vi "Steer towards next Coordinate.vi"(1 "Destination Longitude":dbl=39.689375 format="%#_14g", 2 "Destination Latitude":dbl=-121.824251 format="%#_14g") -> (0 "Steer Value Output String":string)   [LabVIEW 2011]
uses:
  _GlobalVariables&Libraries/ATV Program Global Variables.vi
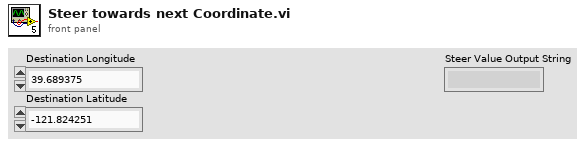
[diagram p1: front panel]
types:
  T1 = cluster{"GPS VISA resource name":refnum<visa-resource-name>, "GPS Error":errorcluster, "Disable GPS VISA":bool, "Latitude":dbl, "Longitude":dbl, "Latitude Uncertainty":dbl, "Longitude Uncertainty":dbl, "GPS Signal":u32}
  T2 = cluster{"Navigation Coordinates":cluster{"Latitude":dbl, "Longitude":dbl}[], "Coordinate Count":u32, "Drive Speed":string, "Steer Angle":dbl, "Steering":dbl, "Direction to next Coordinate":dbl, "Drive":dbl, "Navigation Path":string}
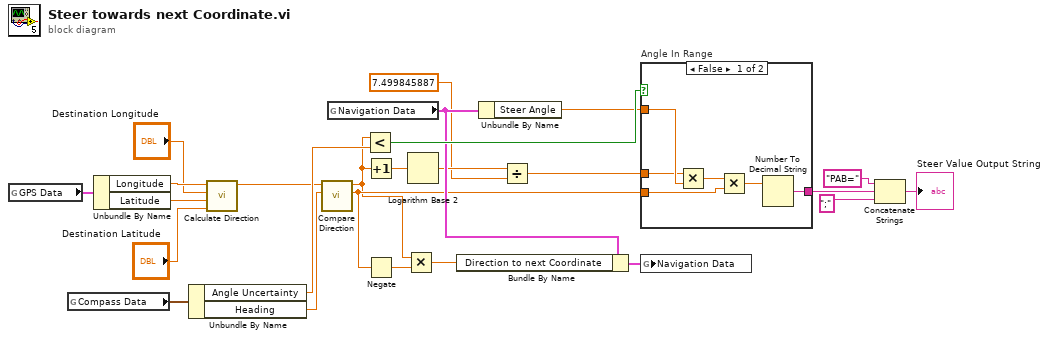
[diagram p0: block diagram]
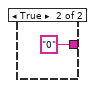
[diagram p2: hidden frame]
diagram:
  n1 = global read "ATV Program Global Variables.vi" "GPS Data"() -> (w18:T1)
  n2 = global read "ATV Program Global Variables.vi" "Compass Data"() -> (w25:cluster{"Angle Uncertainty":dbl, "Heading":dbl})
  n3 = Unbundle By Name(w18) -> ("Longitude"=w17:dbl, "Latitude"=w16:dbl)
  n4 = Unbundle By Name(w25) -> ("Angle Uncertainty"=w24:dbl, "Heading"=w11:dbl)
  n5 = call "Calculate Direction.vi"("Y1"="Destination Latitude", "Y0"=w16, "X1"="Destination Longitude", "X0"=w17) -> ("Destination Bearing"=w10:dbl)  [unwired: 4 in, 3 out]
  n6 = call "Compare Direction.vi"("Current Angle"=w11, "Destination Angle"=w10) -> ("CW(-1)/CCW(1)"=w9:dbl, "Angle to Next Destination"=w2:dbl)  [unwired: 8 in]
  n7 = global read "ATV Program Global Variables.vi" "Navigation Data"() -> (w12:T2)
  n8 = Less?(x=w2, y=w24) -> (x < y?=w23:bool)
  n9 = Increment(x=w2) -> (x+1=w5:dbl)
  n10 = Negate(x=w9) -> (-x=w8:dbl)
  n11 = Multiply(x=w2, y=w8) -> (x*y=w6:dbl)
  n12 = Logarithm Base 2(1:w5) -> (0:w4:dbl)
  n13 = Bundle By Name(cluster=w12, "Direction to next Coordinate"=w6) -> (w13:T2)
  n14 = Unbundle By Name(w12) -> ("Steer Angle"=w7:dbl)
  n15 = Divide(x=w4, y=7.499845887) -> (x/y=w1:dbl)
  n16 = case "Angle In Range" shown="False" w23 {
    tunnel: [w27 "0"] -> w21
    tunnel: w7 -> [w31 _]
    tunnel: w9 -> [w29 _]
    tunnel: w1 -> [w26 _]
    frame False {
      n17 = Multiply(x=w26, y=w31) -> (x*y=w30:dbl)
      n18 = Multiply(x=w30, y=w29) -> (x*y=w28:dbl)
      n19 = Number To Decimal String(number=w28) -> (decimal integer string=w27:string)  [unwired: 1 in]
    }
    frame True {
    }
  }
  n20 = global write "ATV Program Global Variables.vi" "Navigation Data"(w13) -> ()
  n21 = Concatenate Strings("PAB=" ("string"), w21, ";" ("string")) -> (→"Steer Value Output String":string)
